vi "Get_Latest_Newfi.vi"(11 "Error In":errorcluster) -> (4 "Output Path":path, 15 "Error Out 2":errorcluster)   [LabVIEW 2016]
uses:
  <vilib>/Utility/error.llb/Error Cluster From Error Code.vi
  <vilib>/ErrorRing/Error Ring.xnode
  <vilib>/httpClient/LabVIEWHTTPClient.lvlib
  <vilib>/zip/NI_Unzip.lvlib
panel:
  out "File Path Out":string
  out "Status":string
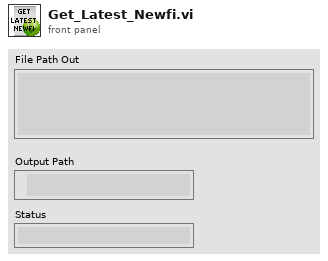
[diagram p1: front panel]
types:
  T1 = typedef "LabVIEWHTTPClient.lvlib/ClientHandle.ctl" = refnum<k1>
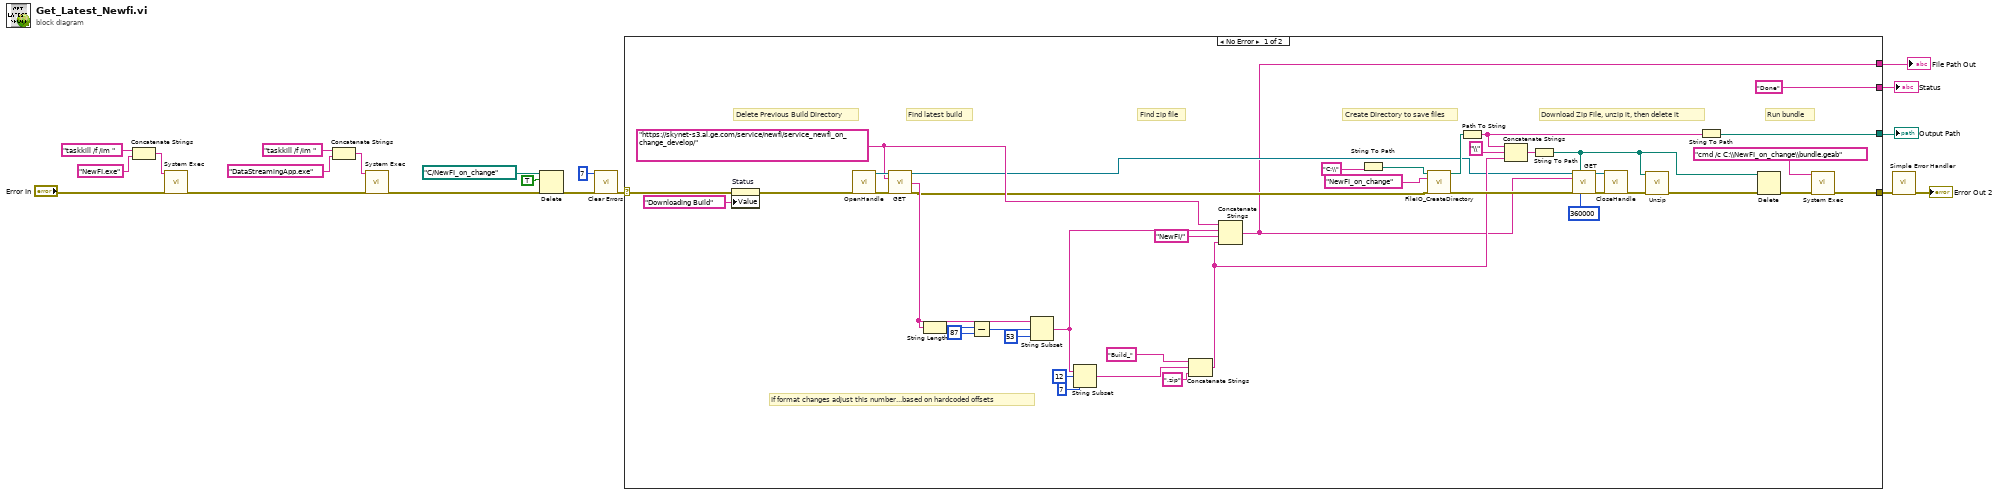
[diagram p0: block diagram]
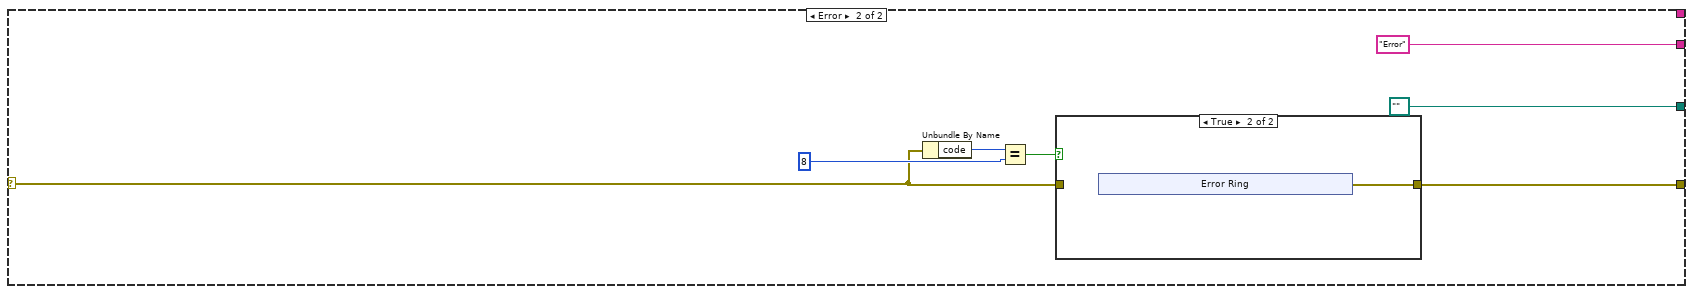
[diagram p2: hidden frame]
diagram:
  n1 = Concatenate Strings("taskkill /f /im " ("string"), "NewFI.exe" ("Task Name")) -> (w6:string)
  n2 = call <vilib>:"System Exec.vi"("error in (no error)"="Error In", "command line"=w6) -> ("error out"=w3:errorcluster)  [unwired: 6 in, 3 out]
  n3 = Concatenate Strings("taskkill /f /im " ("string"), "DataStreamingApp.exe" ("Task Name")) -> (w8:string)
  n4 = call <vilib>:"System Exec.vi"("error in (no error)"=w3, "command line"=w8) -> ("error out"=w7:errorcluster)  [unwired: 6 in, 3 out]
  n5 = Delete(path (use dialog)=path "C:/NewFI_on_change", entire hierarchy (F)=TRUE, error in=w7) -> (error out=w15:errorcluster)  [unwired: 2 in, 2 out]
  n6 = call <vilib>:"Clear Errors.vi"("error in (no error)"=w15, "specific error code to clear (0: all)"=7) -> ("error out"=w14:errorcluster)  [unwired: 4 in, 1 out]
  n7 = case shown="No Error" w14 {
    selector: w14 -> [w37 w62]
    tunnel: [w45 w61] -> w13
    tunnel: [w41 path ""] -> w19
    tunnel: ["Done" "Error"] -> w18
    tunnel: [w20 _] -> w1
    frame No Error {
      w31 = "https://skynet-s3.al.ge.com/service/newfi/service_newfi_on_change_develop/"
      # "If format changes adjust this number...based on hardcoded offsets"
      # "Run bundle"
      # "Delete Previous Build Directory"
      # "Create Directory to save files"
      # "Find zip file"
      # "Find latest build"
      # "Download Zip File, unzip it, then delete it"
      n8 = property on="Status" class="Str"(error in=w37, "Value"="Downloading Build" ("Status")) -> (error out=w38:errorcluster)  [unwired: 1 in, 1 out]
      n9 = call <vilib>:"OpenHandle.vi"("error in (no error)"=w38) -> ("client handle out"=w59:T1, "error out"=w60:errorcluster)  [unwired: 13 in]
      n10 = call <vilib>:"GET.vi"("client handle"=w59, "url"=w31, "error in (no error)"=w60) -> ("client handle out"=w21:T1, "body"=w36:string, "error out"=w29:errorcluster)  [unwired: 9 in, 1 out]
      n11 = String Length(string=w36) -> (length=w35:i32)
      n12 = Subtract(x=w35, y=87) -> (x-y=w33:i32)
      n13 = String Subset(string=w36, offset (0)=w33, length (rest)=53 ("length (rest)")) -> (substring=w28:string)
      n14 = String Subset(string=w28, offset (0)=12, length (rest)=7 ("length (rest)")) -> (substring=w24:string)
      n15 = Concatenate Strings("Build_", w24, ".zip" ("string")) -> (w22:string)
      n16 = Concatenate Strings(w31, w28, "NewFI/" ("Target File Path"), w22) -> (w20:string)
      n17 = String To Path(string="C:\\") -> (path=w47:path)
      n18 = call "FileIO_CreateDirectory.vi"("Base Path"=w47, "Directory Name"="NewFI_on_change", "Error In"=w29) -> ("File Path Control"=w50:path, "Error Out"=w40:errorcluster)  [unwired: 11 in]
      n19 = Path To String(path=w50) -> (string=w44:string)
      n20 = Concatenate Strings(w44, "\\" ("string"), w22) -> (w55:string)
      n21 = String To Path(string=w55) -> (path=w54:path)
      n22 = call <vilib>:"GET.vi"("client handle"=w21, "output file"=w54, "url"=w20, "error in (no error)"=w40, "timeout (10000)"=360000) -> ("client handle out"=w58:T1, "error out"=w57:errorcluster)  [unwired: 7 in, 2 out]
      n23 = call <vilib>:"CloseHandle.vi"("client handle"=w58, "error in (no error)"=w57) -> ("error out"=w51:errorcluster)  [unwired: 13 in]
      n24 = call <vilib>:"Unzip.vi"("error in (no error)"=w51, "Zip file"=w54) -> ("error out"=w53:errorcluster)  [unwired: 7 in, 2 out]
      n25 = String To Path(string=w44) -> (path=w41:path)
      n26 = Delete(path (use dialog)=w54, error in=w53) -> (error out=w46:errorcluster)  [unwired: 3 in, 2 out]
      n27 = call <vilib>:"System Exec.vi"("error in (no error)"=w46, "command line"="cmd /c C:\\NewFI_on_change\\bundle.geab" ("string")) -> ("error out"=w45:errorcluster)  [unwired: 6 in, 3 out]
    }
    frame Error {
      n28 = Unbundle By Name(w62) -> ("code"=w66:i32)
      n29 = Equal?(x=w66, y=8) -> (x = y?=w63:bool)
      n30 = case shown="True" w63 {
        tunnel: w62 -> [w68 _]
        tunnel: [w68 w69] -> w61
        frame False {
        }
        frame True {
          n31 = xnode "Error Ring"() -> ("error out"=w69:errorcluster)
        }
      }
    }
  }
  "Output Path" <- w19
  "Status" <- w18
  "File Path Out" <- w1
  n32 = call <vilib>:"Simple Error Handler.vi"("error in (no error)"=w13) -> ("error out"=→"Error Out 2":errorcluster)  [unwired: 4 in, 4 out]
